vi "Continue Compute Path.vi"(11 "AD* in":refnum<class "NI_Robotics_AnytimeDStar.lvclass">) -> (2 "continue computing path":bool, 3 "AD* out":refnum<class "NI_Robotics_AnytimeDStar.lvclass">)   [LabVIEW 2017, in "NI_Robotics_AnytimeDStar.lvclass"]
uses:
  <vilib>/robotics/Navigation/Anytime D Star/NI_Robotics_AnytimeDStar.lvclass
  <vilib>/robotics/Navigation/Anytime D Star/NI_Robotics_AnytimeDStar.lvclass/NI_Robotics_AnytimeDStar.ctl
  <vilib>/robotics/Navigation/shared/MapNode/AbstractDstarNode/NI_Robotics_AbstractDstarNode.lvclass
  <vilib>/robotics/Navigation/shared/Priority Queue/NI_Robotics_Priority Queue.lvclass
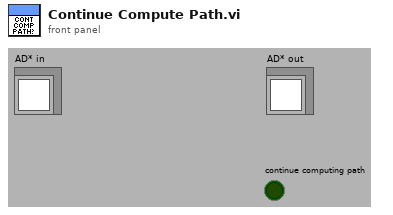
[diagram p1: front panel]
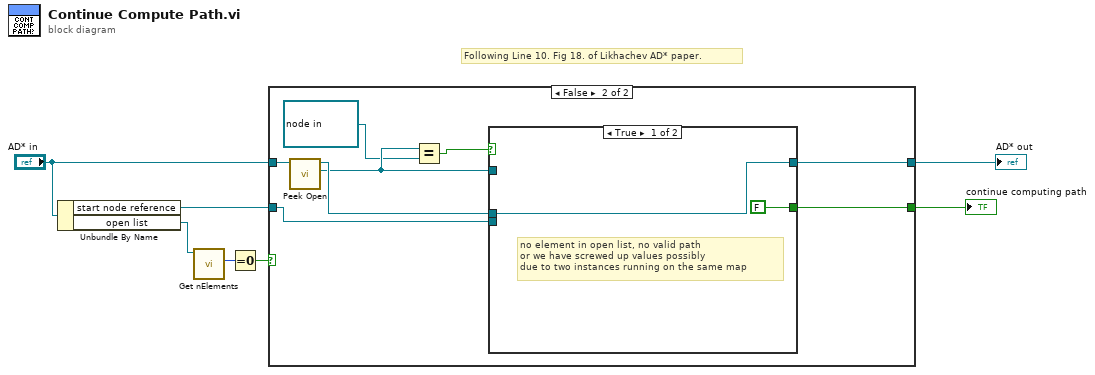
[diagram p0: block diagram]
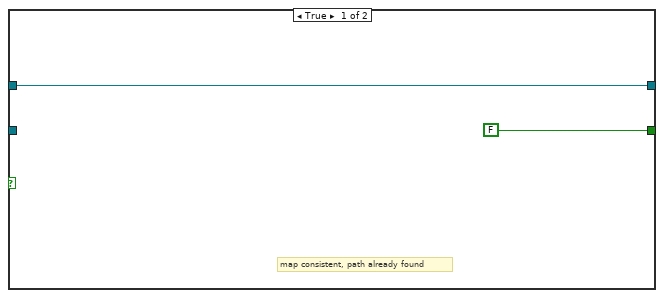
[diagram p2: hidden frame]
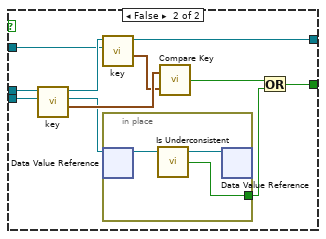
[diagram p3: hidden frame]
diagram:
  # "Following Line 10. Fig 18. of Likhachev AD* paper."
  n1 = Unbundle By Name("AD* in") -> ("start node reference"=w6:refnum<data-value>, "open list"=w4:refnum<class "NI_Robotics_Priority Queue.lvclass">)
  n2 = call <vilib>:"Get nElements.vi"("Priority Queue in"=w4) -> ("nElements"=w3:i32)  [unwired: 9 in, 1 out]
  n3 = Equal To 0?(x=w3) -> (x = 0?=w2:bool)
  n4 = case shown="False" w2 {
    tunnel: [FALSE w17] -> w7
    tunnel: w6 -> [_ w10]
    tunnel: "AD* in" -> [w8 w16]
    tunnel: [w8 w14] -> w1
    frame True {
      # "map consistent, path already found"
    }
    frame False {
      n5 = call <vilib>:"Peek Open.vi"("adstar in"=w16) -> ("node ref out"=w13:refnum<data-value>, "adstar out"=w15:refnum<class "NI_Robotics_AnytimeDStar.lvclass">)  [unwired: 9 in]
      n6 = Equal?(x=w13, y=refnum<data-value> refnum) -> (x = y?=w11:bool)
      n7 = case shown="True" w11 {
        tunnel: [FALSE w30] -> w17
        tunnel: w10 -> [_ w24]
        tunnel: w15 -> [w18 w22]
        tunnel: [w18 w21] -> w14
        tunnel: w13 -> [_ w20]
        frame True {
          # "no element in open list, no valid path\nor we have screwed up values possibly\ndue to two instances running on the same map"
        }
        frame False {
          n8 = call <vilib>:"key.vi"("node ref in"=w24, "adstar in"=w22) -> ("key out"=w29:cluster{"(g or v) + h":dbl, "g or v":dbl}, "node ref out"=w23:refnum<data-value>, "adstar out"=w27:refnum<class "NI_Robotics_AnytimeDStar.lvclass">)  [unwired: 7 in]
          n9 = call <vilib>:"key.vi"("node ref in"=w20, "adstar in"=w27) -> ("key out"=w28:cluster{"(g or v) + h":dbl, "g or v":dbl}, "adstar out"=w21:refnum<class "NI_Robotics_AnytimeDStar.lvclass">)  [unwired: 7 in, 1 out]
          n10 = in-place {
            in-place-border: [w31] -> w26
            n11 = in-place-dvr #1(w23) -> (w32:refnum<class "NI_Robotics_AbstractDstarNode.lvclass">)  [unwired: 1 out]
            n12 = call <vilib>:"Is Underconsistent.vi"("AbstractDstarNode in"=w32) -> ("is Underconsistent"=w31:bool, "AbstractDstarNode out"=w33:refnum<class "NI_Robotics_AbstractDstarNode.lvclass">)  [unwired: 2 in, 1 out]
            n13 = in-place-dvr #1(w33) -> ()  [unwired: 2 out]
          }
          n14 = call <vilib>:"Compare Key.vi"("keyB in"=w28, "keyA in"=w29) -> ("keyA > keyB"=w25:bool)
          n15 = Or(x=w25, y=w26) -> (x .or. y?=w30:bool)
        }
      }
    }
  }
  "continue computing path" <- w7
  "AD* out" <- w1
